vi "FTW-Actor-Destroy.vi"(0 "FTW Actor Instance":refnum<class "FTW-ActorInstance.lvclass">, 5 "Force Destroy?":bool=TRUE, 11 "error in":errorcluster) -> (15 "error out":errorcluster)   [LabVIEW 2012, in "FTW-Actor.lvlib" / "FTW-ActorInstance.lvclass"]
uses:
  FTW-ActorInstance.lvclass
  FTW-ActorInstance.lvclass/FTW-ActorInstance.ctl
  Endpoint/FTW-Endpoint.lvclass
  JobSequencer/FTW-JobSequencer.lvclass
panel:
  # "Inputs"
  # "Outputs"
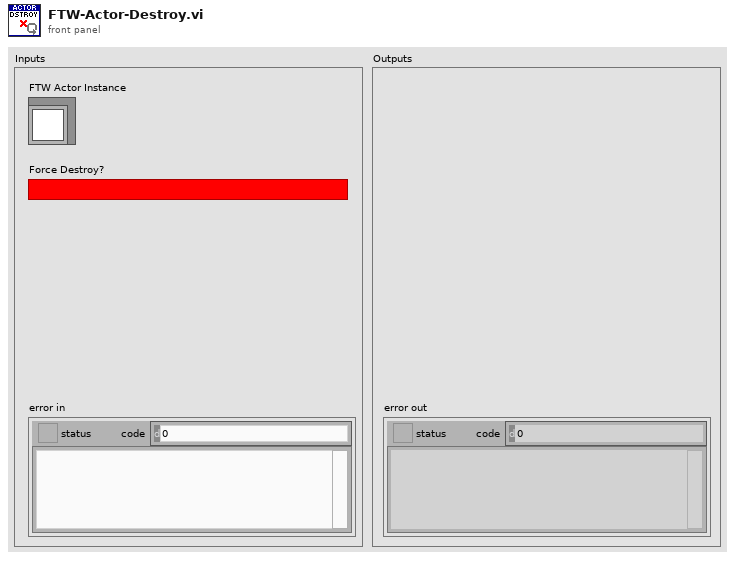
[diagram p1: front panel]
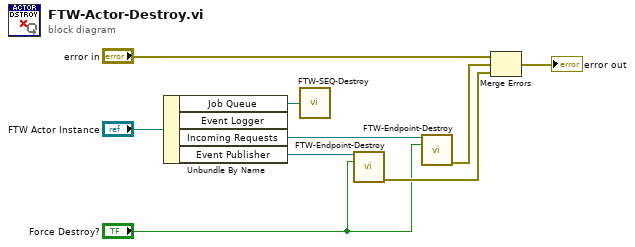
[diagram p0: block diagram]
diagram:
  n1 = Unbundle By Name("FTW Actor Instance") -> ("Job Queue"=w6:refnum<class "FTW-JobSequencer.lvclass">, "Incoming Requests"=w4:refnum<class "FTW-Endpoint.lvclass">, "Event Publisher"=w3:refnum<class "FTW-Endpoint.lvclass">)  [unwired: 1 out]
  n2 = call "FTW-SEQ-Destroy.vi"("Sequencer"=w6) -> ()  [unwired: 1 in]
  n3 = call-dynamic "FTW-Endpoint-Destroy.vi"("FTW Endpoint Type"=w3, "Force Destroy"="Force Destroy?") -> ("error out"=w2:errorcluster)  [unwired: 13 in]
  n4 = call-dynamic "FTW-Endpoint-Destroy.vi"("FTW Endpoint Type"=w4, "Force Destroy"="Force Destroy?") -> ("error out"=w5:errorcluster)  [unwired: 13 in]
  n5 = Merge Errors("error in", w5, w2) -> (→"error out":errorcluster)
